vi "Silhouette_Score.vi"(8 "error in (no error)":errorcluster caption="entrée d'erreur (pas d'erreur)", 9 "labels":string[][](array[string]), 10 "X":string[][](array[string]), 11 "silhouette_score":T1={"metric"="euclidean", "sample_size"="None", "random_state"=-1} {"random_state" min=-1}) -> (0 "error out":errorcluster caption="sortie d'erreur", 3 "Score":string)   [LabVIEW 2020]
doc: "Compute the mean Silhouette Coefficient of all samples.\n\nThe Silhouette Coefficient is calculated using the mean intra-cluster distance (a) and the mean nearest-cluster distance (b) for each sample. The Silhouette Coefficient for a sample is (b - a) / max(a, b). To clarify, b is the distance between a sample and the nearest cluster that the sample is not a part of. Note that Silhouette Coefficient is only defined if number of labels is 2 <= n_labels <= n_samples - 1.\n\nThis function returns the mean Silhouette Coefficient over all samples. To obtain the values for each sample, use silhouette_samples.\n\nThe best value is 1 and the worst value is -1. Values near 0 indicate overlapping clusters. Negative values generally indicate that a sample has been assigned to the wrong cluster, as a different cluster is more similar.\n\n\n\nParameters : \n\n- X : array [n_samples_a, n_samples_a] if metric == “precomputed”, or, [n_samples_a, n_features] otherwise\nArray of pairwise distances between samples, or a feature array.\n\n- labels : array, shape = [n_samples]\nPredicted labels for each sample.\n\n- metric : string, or callable\nThe metric to use when calculating distance between instances in a feature array. If metric is a string, it must be one of the options allowed by metrics.pairwise.pairwise_distances. If X is the distance array itself, use metric=\"precomputed\".\n\n- sample_size : int or None\nThe size of the sample to use when computing the Silhouette Coefficient on a random subset of the data. If sample_size is None, no sampling is used.\n\n- random_state : int, RandomState instance or None, optional (default=None=-1)\nDetermines random number generation for selecting a subset of samples. Used when sample_size is not None. Pass an int for reproducible results across multiple function calls. See Glossary.\n\nReturns : \n\n- silhouette : float\nMean Silhouette Coefficient for all samples."
uses:
  Silhouette_Score.lvclass
panel:
  out "Silhouette_Score.lvclass":refnum<class "Silhouette_Score.lvclass">
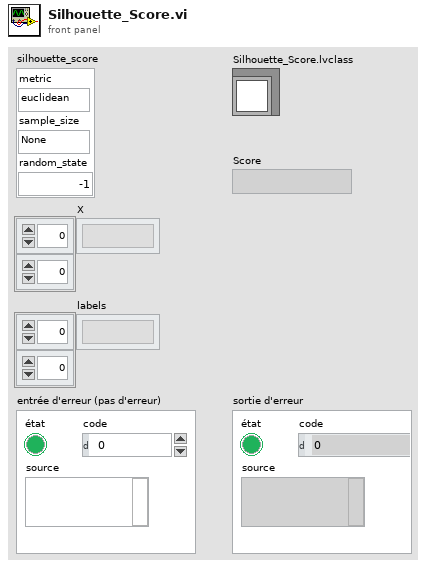
[diagram p1: front panel]
types:
  T1 = cluster{"metric":string, "sample_size":string, "random_state":i32}
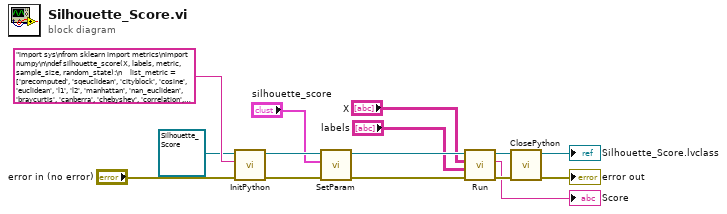
[diagram p0: block diagram]
diagram:
  n1 = call-dynamic "InitPython.vi"("error in (no error)"="error in (no error)", "Python Instruction"="import sys\nfrom sklearn import metrics\nimport numpy\n\ndef silhouette_score(X, labels, metric, sample_size, random_state):\n    list_metric = ['precomputed', 'sqeuclidean', 'cityblock', 'cosine', 'euclidean', 'l1', 'l2', 'manhattan', 'nan_euclidean', 'braycurtis', 'canberra', 'chebyshev', 'correlation', 'dice', 'hamming', 'jaccard', 'kulsinski', 'mahalanobis', 'minkowski', 'rogerstanimoto', 'russellrao', 'seuclidean', 'sokalmichener', 'sokalsneath', 'sqeuclidean', 'yule']\n    X = eval(X)\n    labels = eval(labels)\n    if metric not in list_metric:\n        metric = eval(metric) \n    if sample_size == 'None':\n        sample_size = None\n    if random_state == -1:\n        random_state = None\n    try:\n        silhouette_score = metrics.silhouette_score(X, labels, metric, sample_size, random_state)\n        silhouette_score = silhouette_score.tolist()\n        return str(silhouette_score)\n    except:\n        erreur = sys.exc_info()\n        typerr = u\"%s\" % (erreur[0])\n        typerr = typerr[typerr.find(\"'\")+1:typerr.rfind(\"'\")]\n        msgerr = u\"%s\" % (erreur[1])\n        message = str('/!\\\\ {0} : {1}'. format(typerr,msgerr))\n        return message", "Scikit-learn en entrée"=refnum<class "Silhouette_Score.lvclass"> refnum ("Silhouette_Score.lvclass")) -> ("error out"=w11:errorcluster, "Scikit-learn en sortie"=w10:refnum<class "Silhouette_Score.lvclass">)  [unwired: 7 in]
  n2 = call-dynamic "SetParam.vi"("error in (no error)"=w11, "silhouette_score"="silhouette_score", "Silhouette_Score.lvclass"=w10) -> ("error out"=w8:errorcluster, "Silhouette_Score.lvclass"=w7:refnum<class "Silhouette_Score.lvclass">)  [unwired: 7 in]
  n3 = call-dynamic "Run.vi"("error in (no error)"=w8, "labels"="labels", "X"="X", "Silhouette_Score.lvclass"=w7) -> ("error out"=w6:errorcluster, "String Data"=→"Score":string, "Silhouette_Score.lvclass"=w5:refnum<class "Silhouette_Score.lvclass">)  [unwired: 5 in]
  n4 = call-dynamic "ClosePython.vi"("error in (no error)"=w6, "Scikit-learn en entrée"=w5) -> ("error out"=→"error out":errorcluster, "Scikit-learn en sortie"=→"Silhouette_Score.lvclass":refnum<class "Silhouette_Score.lvclass">)  [unwired: 8 in]
